vi "D Save and Recall.vi"(6 "operation(Recall:0)":u16(ring) items=["Recall", "Save", "Clear"], 7 "register(1)":i16=1, 8 "error in (no error)":errorcluster, 11 "VISA resource name":refnum<visa-resource-name>) -> (0 "error out":errorcluster, 3 "VISA resource name out":refnum<visa-resource-name>)   [LabVIEW 2018, in "Agilent 87XX Series.lvlib"]
doc: "This function saves and recalls instrument settings and programs to or from registers inside the 8753D. Note: this VI only works for the 8753D."
uses:
  Agilent 87XX Series.lvlib
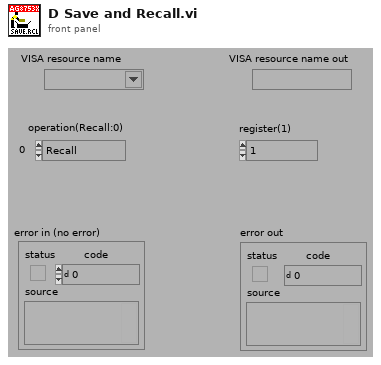
[diagram p1: front panel]
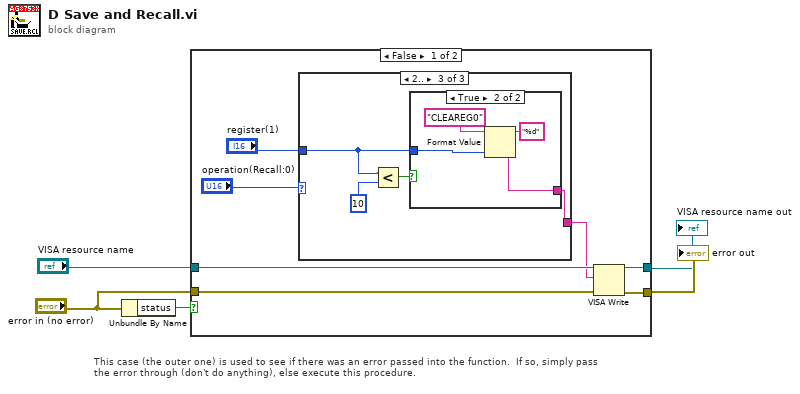
[diagram p0: block diagram]
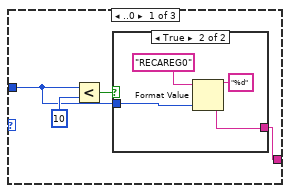
[diagram p2: hidden frame]
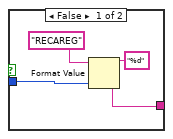
[diagram p3: hidden frame]
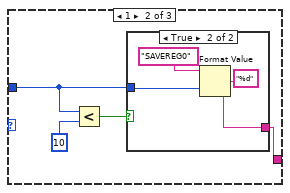
[diagram p4: hidden frame]
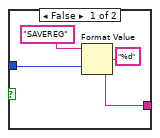
[diagram p5: hidden frame]
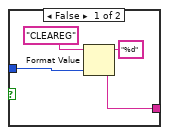
[diagram p6: hidden frame]
diagram:
  # "This case (the outer one) is used to see if there was an error passed into the function.  If so, simply pass \nthe error through (don't do anything), else execute this procedure."
  n1 = Unbundle By Name("error in (no error)") -> ("status"=w5:bool)
  n2 = case shown="False" w5 {
    tunnel: [w12 w49] -> w3
    tunnel: "VISA resource name" -> [w11 w50]
    tunnel: [w10 w50] -> w1
    tunnel: "error in (no error)" -> [w7 w49]
    frame False {
      n3 = case shown="2.." "operation(Recall:0)" {
        tunnel: "register(1)" -> [w13 w25 w37]
        tunnel: [w16 w28 w40] -> w6
        frame ..0 {
          n4 = Less?(x=w13, y=i16 10) -> (x < y?=w14:bool)
          n5 = case shown="True" w14 {
            tunnel: [w19 w23] -> w16
            tunnel: w13 -> [w17 w21]
            frame False {
              n6 = Format Value(string ("")="RECAREG", format string="%d", value (0)=w17) -> (output string=w19:string)
            }
            frame True {
              n7 = Format Value(string ("")="RECAREG0", format string="%d", value (0)=w21) -> (output string=w23:string)
            }
          }
        }
        frame 1 {
          n8 = Less?(x=w25, y=i16 10) -> (x < y?=w26:bool)
          n9 = case shown="True" w26 {
            tunnel: w25 -> [w32 w36]
            tunnel: [w31 w35] -> w28
            frame False {
              n10 = Format Value(string ("")="SAVEREG", format string="%d", value (0)=w32) -> (output string=w31:string)
            }
            frame True {
              n11 = Format Value(string ("")="SAVEREG0", format string="%d", value (0)=w36) -> (output string=w35:string)
            }
          }
        }
        frame 2.. {
          n12 = Less?(x=w37, y=i16 10) -> (x < y?=w38:bool)
          n13 = case shown="True" w38 {
            tunnel: [w44 w48] -> w40
            tunnel: w37 -> [w43 w47]
            frame False {
              n14 = Format Value(string ("")="CLEAREG", format string="%d", value (0)=w43) -> (output string=w44:string)
            }
            frame True {
              n15 = Format Value(string ("")="CLEAREG0", format string="%d", value (0)=w47) -> (output string=w48:string)
            }
          }
        }
      }
      n16 = VISA Write(VISA resource name=w11, write buffer=w6, error in (no error)=w7) -> (VISA resource name out=w10:refnum<visa-resource-name>, error out=w12:errorcluster)  [unwired: 1 out]
    }
    frame True {
    }
  }
  "error out" <- w3
  "VISA resource name out" <- w1
